vi "Parse Numbers.vi"(11 "string array":string[](array[string])) -> (3 "Array":refnum<class "Number.lvclass">[](array[class]))   [LabVIEW 2020, in "Schema Parser.lvclass"]
uses:
  Schema Parser.lvclass
  Number/Number.lvclass
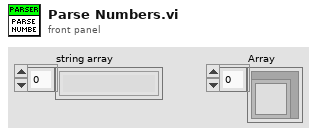
[diagram p1: front panel]
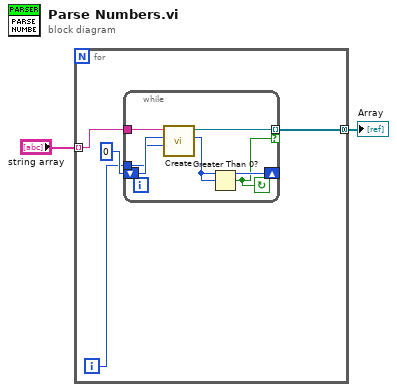
[diagram p0: block diagram]
diagram:
  n1 = for {
    tunnel: "string array" -> [w6] mode=indexing
    tunnel: [w3] -> w2 mode=concatenating
    i -> [w4]
    n2 = while {
      tunnel: w6 -> [w12]
      tunnel: [w11] -> w3 mode=indexing if=w7
      tunnel: w4 -> [w9]
      shift-right: [w8] -> _
      shift-left: 0 ("Col Offset") -> [w10]
      stop <- w7 continue-if-true
      n3 = call "Create.vi"("Row"=w9, "Col Offset"=w10, "String"=w12) -> ("Offset Past Number"=w8:i32, "Number"=w11:refnum<class "Number.lvclass">)  [unwired: 6 in, 1 out]
      n4 = Greater Than 0?(x=w8) -> (x > 0?=w7:bool)
    }
  }
  "Array" <- w2
